vi "test.vi"() -> ()   [LabVIEW 2017]
panel:
  out "output cluster":cluster{cluster{"Scalar":dbl}[]}
  out "appended array":cluster{"Scalar":dbl}[][](array[cluster])
  in  "stop":bool
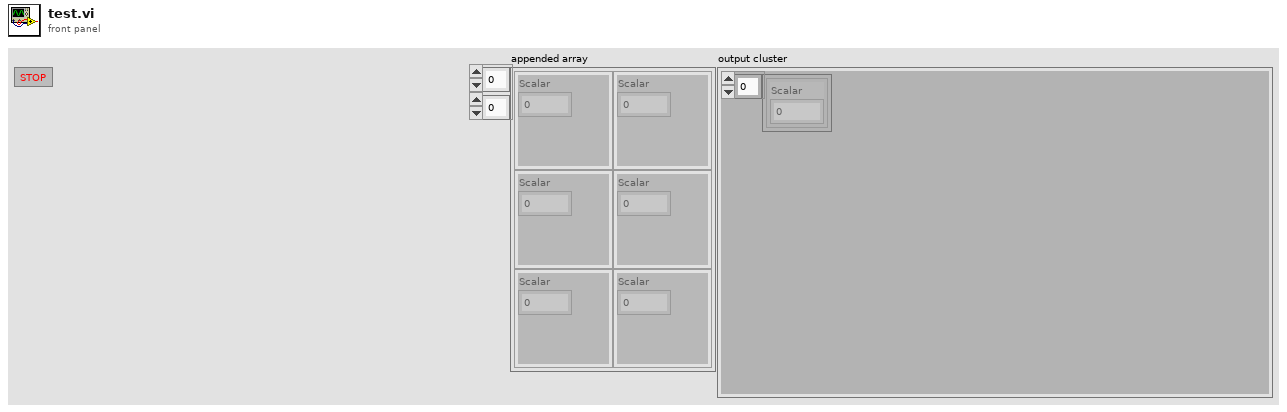
[diagram p1: front panel]
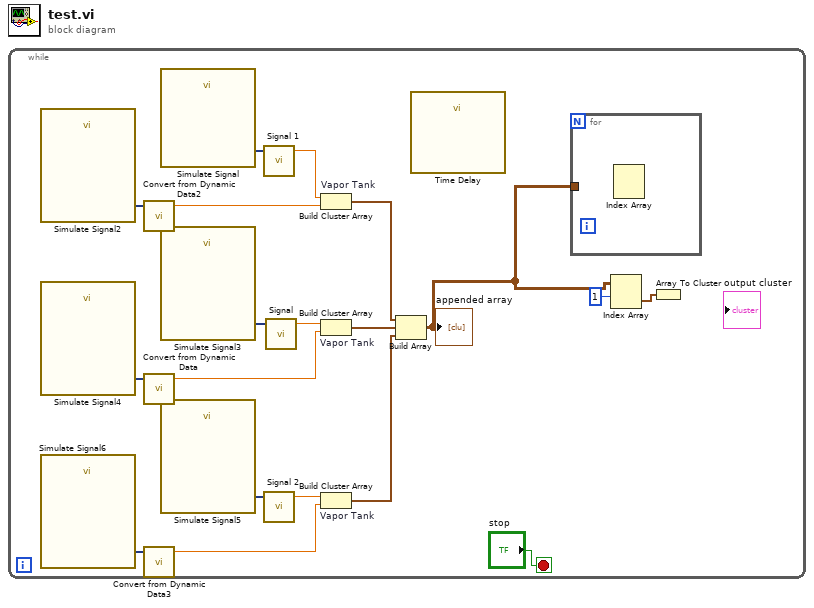
[diagram p0: block diagram]
diagram:
  n1 = while {
    stop <- "stop" stop-if-true
    n2 = call "Simulate Signal2"() -> ("Sine"=w18:dynamicdata)  [unwired: 14 in, 1 out]
    n3 = call "Simulate Signal4"() -> ("Sine"=w12:dynamicdata)  [unwired: 14 in, 1 out]
    n4 = call "Simulate Signal6"() -> ("Sine"=w7:dynamicdata)  [unwired: 14 in, 1 out]
    n5 = call "Convert from Dynamic Data2"("Dynamic Data Type"=w18) -> ("Scalar"=w16:dbl)  [unwired: 3 in]
    n6 = call "Convert from Dynamic Data"("Dynamic Data Type"=w12) -> ("Scalar"=w14:dbl)  [unwired: 3 in]
    n7 = call "Convert from Dynamic Data3"("Dynamic Data Type"=w7) -> ("Scalar"=w5:dbl)  [unwired: 3 in]
    n8 = call "Simulate Signal"() -> ("Sine"=w19:dynamicdata)  [unwired: 14 in, 1 out]
    n9 = call "Simulate Signal3"() -> ("Sine"=w11:dynamicdata)  [unwired: 14 in, 1 out]
    n10 = call "Simulate Signal5"() -> ("Sine"=w8:dynamicdata)  [unwired: 14 in, 1 out]
    n11 = call "Signal 1"("Dynamic Data Type"=w19) -> ("Scalar"=w17:dbl)  [unwired: 3 in]
    n12 = call "Signal 2"("Dynamic Data Type"=w8) -> ("Scalar"=w6:dbl)  [unwired: 3 in]
    n13 = call "Signal"("Dynamic Data Type"=w11) -> ("Scalar"=w13:dbl)  [unwired: 3 in]
    n14 = Build Cluster Array "Vapor Tank"(w17, w16) -> (w10:cluster{"Scalar":dbl}[])
    n15 = Build Cluster Array "Vapor Tank"(w13, w14) -> (w9:cluster{"Scalar":dbl}[])
    n16 = Build Cluster Array "Vapor Tank"(w6, w5) -> (w4:cluster{"Scalar":dbl}[])
    n17 = Build Array(w10, w9, w4) -> (w3:cluster{"Scalar":dbl}[][])
    "appended array" <- w3
    n18 = call "Time Delay"() -> ()  [unwired: 11 in, 1 out]
    n19 = for {
      tunnel: w3 -> [_]
      n20 = Index Array() -> ()  [unwired: 3 in, 1 out]
    }
    n21 = Index Array(array=w3, index (row)=1) -> (element=w1:cluster{"Scalar":dbl}[])  [unwired: 1 in]
    n22 = Array To Cluster(array=w1) -> ()  [unwired: 1 out]
  }
